vi "加标回收参数设置.vi"() -> ()   [LabVIEW 2016, in "质控单元V1.lvlib"]
panel:
  in  "显示详细日志":bool
  in  "布尔":bool
  in  "Tab Control 2":enum32{"氨氮", "总磷", "总氮", "高锰酸盐指数", "化学需氧量"}(tab)
  in  "启用":bool
  out "氨氮加标回收率":sgl caption="加标回收率" format="%#.2f"
  out "氨氮加标体积":sgl caption="加标体积" format="%#.4f"
  in  "氨氮母液浓度":sgl caption="母液浓度"
  in  "氨氮定容体积":sgl caption="定容体积"
  out "氨氮加标后水样浓度":sgl caption="加标后水样浓度" format="%#.4f"
  out "氨氮加标前水样浓度":sgl caption="加标前水样浓度" format="%#.4f"
  in  "氨氮量程":sgl caption="量程"
  in  "氨氮检出限":sgl caption="检出限"
  in  "启用 2":bool
  out "TP加标回收率":sgl caption="加标回收率" format="%#.2f"
  out "TP加标体积":sgl caption="加标体积" format="%#.4f"
  in  "TP母液浓度":sgl caption="母液浓度"
  in  "TP定容体积":sgl caption="定容体积"
  out "TP加标后水样浓度":sgl caption="加标后水样浓度" format="%#.4f"
  out "TP加标前水样浓度":sgl caption="加标前水样浓度" format="%#.4g"
  in  "TP量程":sgl caption="量程"
  in  "TP检出限":sgl caption="检出限"
  in  "启用 3":bool
  out "TN加标回收率":sgl caption="加标回收率" format="%#.2f"
  out "TN加标体积":sgl caption="加标体积" format="%#.4f"
  in  "TN母液浓度":sgl caption="母液浓度"
  in  "TN定容体积":sgl caption="定容体积"
  out "TN加标后水样浓度":sgl caption="加标后水样浓度" format="%#.4f"
  out "TN加标前水样浓度":sgl caption="加标前水样浓度" format="%#.4f"
  in  "TN量程":sgl caption="量程"
  in  "TN检出限":sgl caption="检出限"
  in  "启用 4":bool
  out "CODMn加标回收率":sgl caption="加标回收率" format="%#.2f"
  out "CODMn加标体积":sgl caption="加标体积" format="%#.4f"
  in  "CODMn母液浓度":sgl caption="母液浓度"
  in  "CODMn定容体积":sgl caption="定容体积"
  out "CODMn加标后水样浓度":sgl caption="加标后水样浓度" format="%#.4f"
  out "CODMn加标前水样浓度":sgl caption="加标前水样浓度" format="%#.4f"
  in  "CODMn量程":sgl caption="量程"
  in  "CODMn检出限":sgl caption="检出限"
  in  "启用 5":bool
  out "CODCr加标回收率":sgl caption="加标回收率" format="%#.2f"
  out "CODCr加标体积":sgl caption="加标体积" format="%#.4f"
  in  "CODCr母液浓度":sgl caption="母液浓度"
  in  "CODCr定容体积":sgl caption="定容体积"
  out "CODCr加标后水样浓度":sgl caption="加标后水样浓度" format="%#.4f"
  out "CODCr加标前水样浓度":sgl caption="加标前水样浓度" format="%#.4f"
  in  "CODCr量程":sgl caption="量程"
  in  "CODCr检出限":sgl caption="检出限"
  # "加标回收参数设置"
  # "加标回收参数"
  # "加标回收参数"
  # "加标回收参数"
  # "加标回收参数"
  # "加标回收参数"
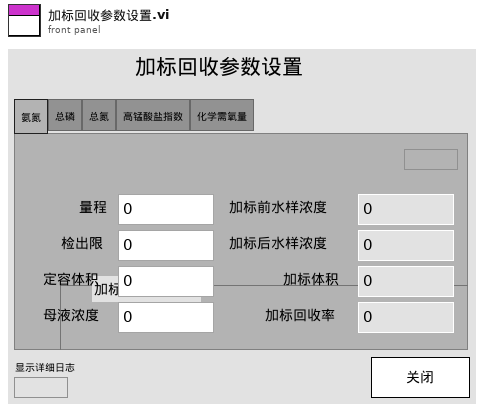
[diagram p1: front panel]
types:
  T1 = cluster{"量程":dbl, "检出限":dbl, "加标前水样浓度":dbl, "加标后水样浓度":dbl, "加标水杯定容体积":dbl, "加标母液浓度":dbl, "加标体积":dbl, "加标回收率":dbl}
  T2 = cluster{"氨氮":bool, "总磷":bool, "总氮":bool, "CODMn":bool, "CODCr":bool, "氨氮总磷":bool, "总磷总氮":bool}
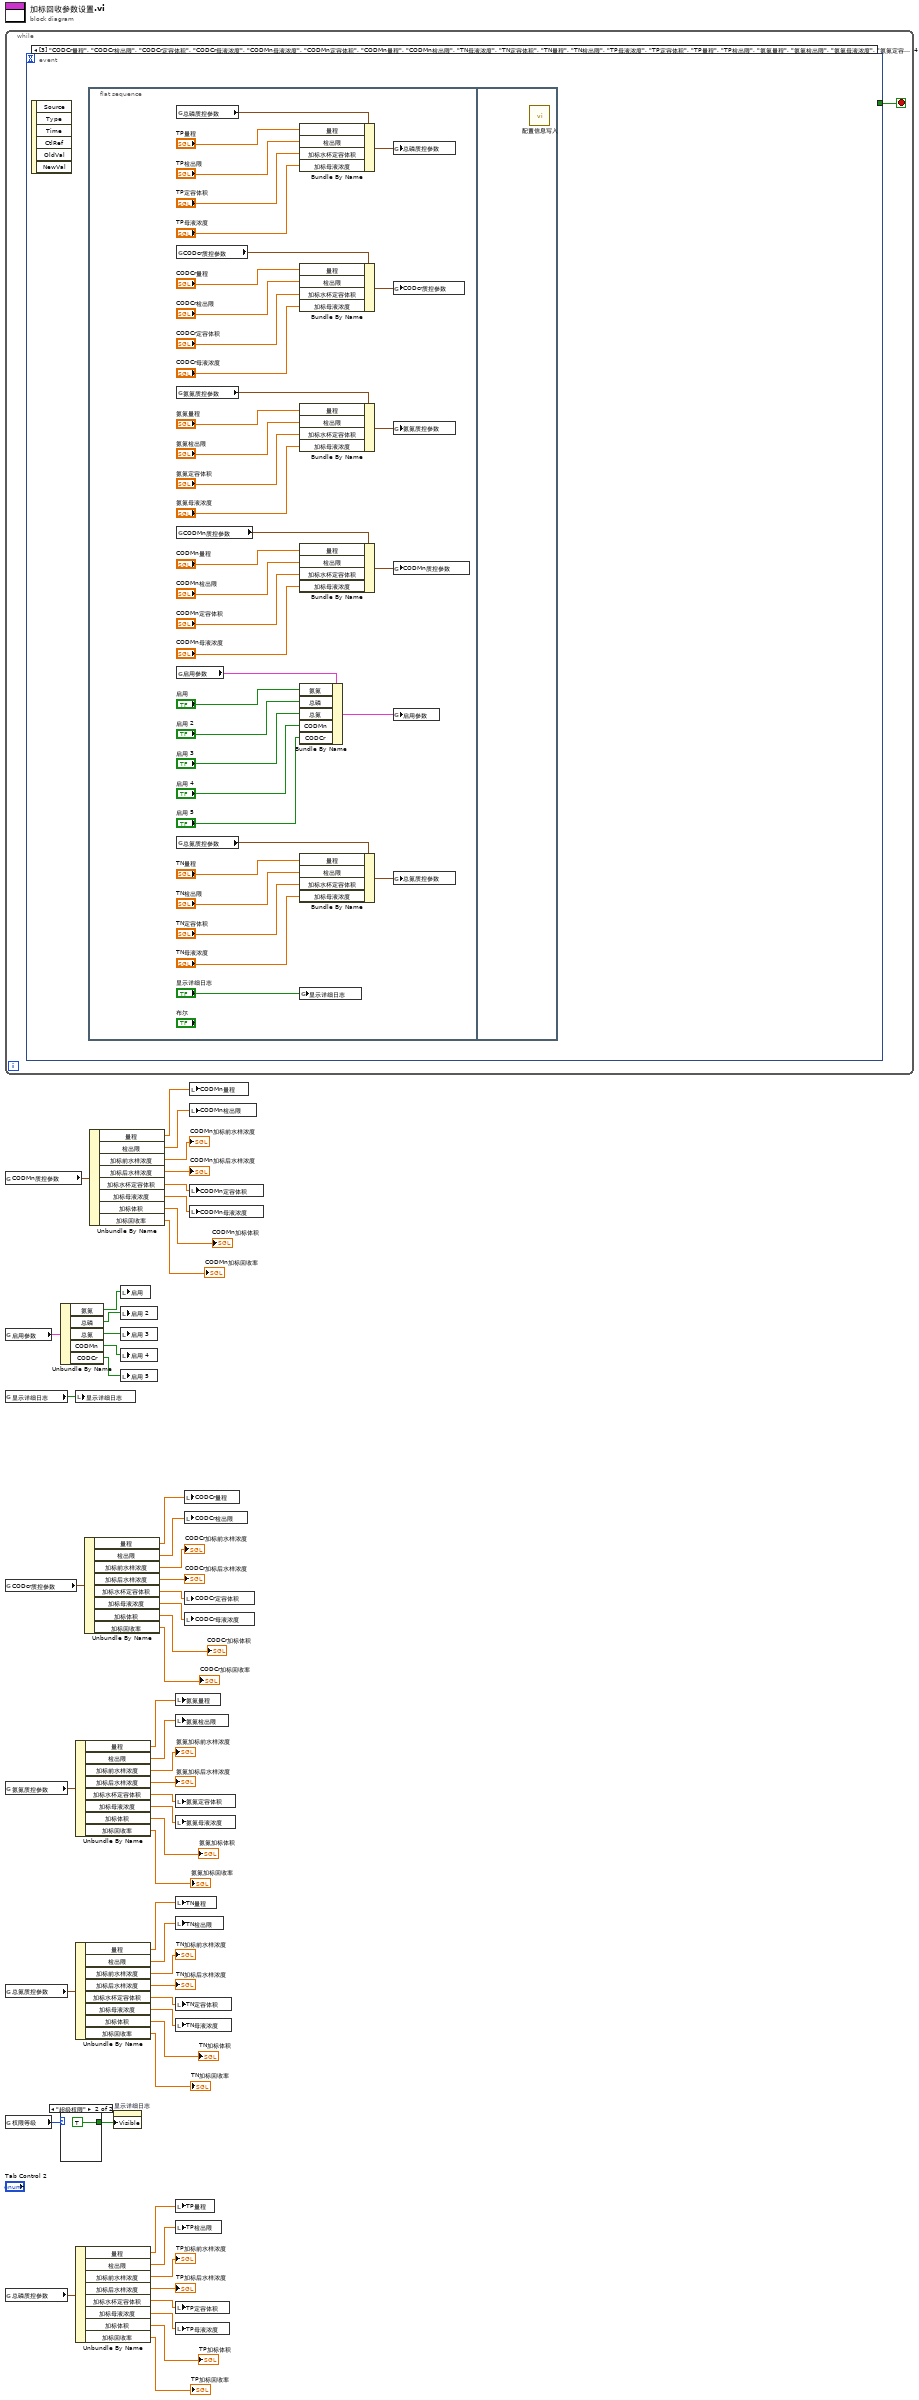
[diagram p0: block diagram]
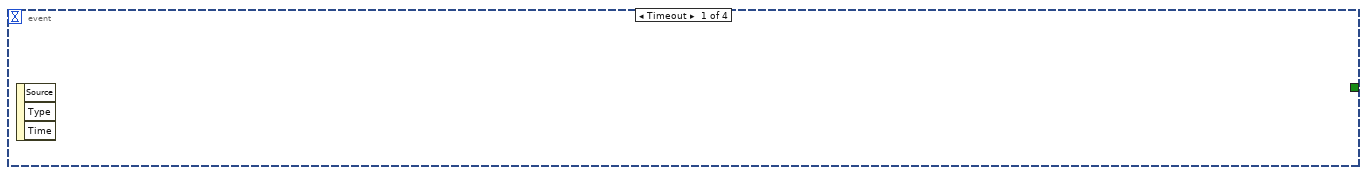
[diagram p3: hidden frame]
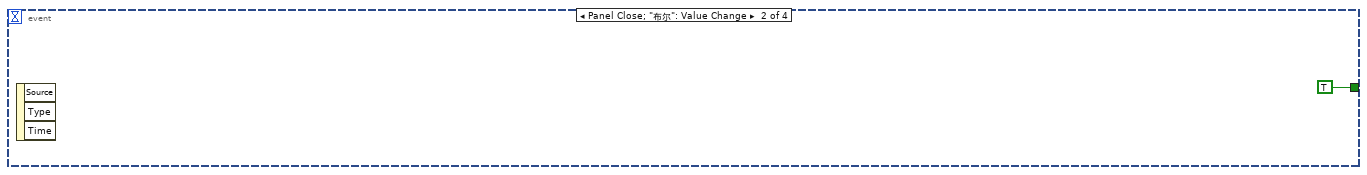
[diagram p4: hidden frame]
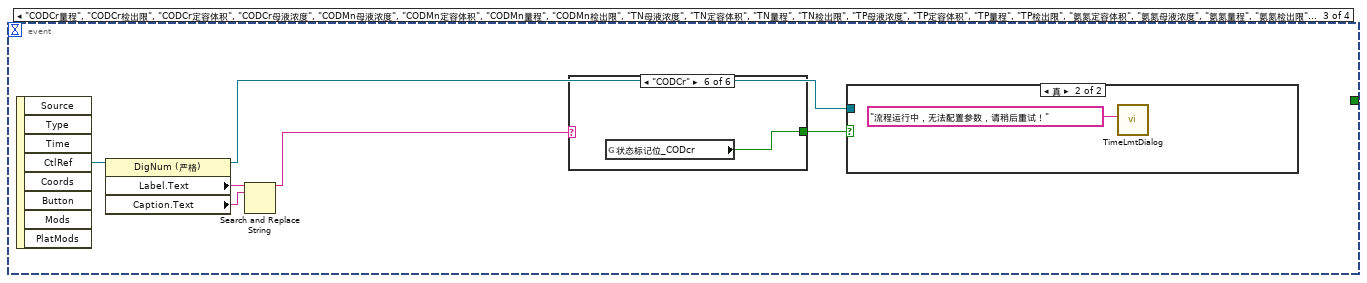
[diagram p5: hidden frame]
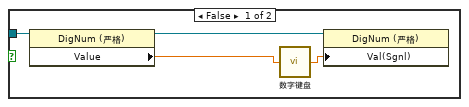
[diagram p6: hidden frame]
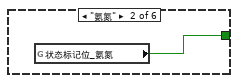
[diagram p8: hidden frame]
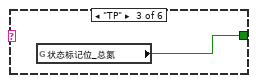
[diagram p9: hidden frame]
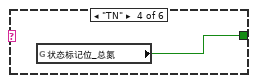
[diagram p10: hidden frame]
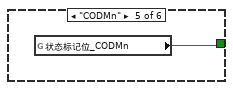
[diagram p11: hidden frame]
diagram:
  n1 = while {
    stop <- w55 stop-if-true
    n2 = event shown="[3] \"CODCr量程\", \"CODCr检出限\", \"CODCr定容体积\", \"CODCr母液浓度\", \"CODMn母液浓度\", \"CODMn定容体积\", \"CODMn量程\", \"CODMn检出限\", \"TN母液浓度\", \"TN定容体积\", \"TN量程\", \"TN检出限\", \"TP母液浓度\", \"TP定容体积\", \"TP量程\", \"TP检出限\", \"氨氮量程\", \"氨氮检出限\", \"氨氮母液浓度\", \"氨氮定容体积\", \"启用\", \"启用 2\", \"启用 3\", \"启用 4\", \"启用 5\", \"显示详细日志\": 值改变" {
      selector: _ -> [_ _ _ _]
      dyn-events: _ -> [_ _ _ _]
      timeout: _ -> [_ _ _ _]
      tunnel: [_ TRUE _ _] -> w55
      event Timeout {
        n3 = event-data() -> ()  [unwired: 1 in, 3 out]
      }
      event Panel Close; "布尔": Value Change {
        n4 = event-data() -> ()  [unwired: 1 in, 3 out]
      }
      event "CODCr量程", "CODCr检出限", "CODCr定容体积", "CODCr母液浓度", "CODMn母液浓度", "CODMn定容体积", "CODMn量程", "CODMn检出限", "TN母液浓度", "TN定容体积", "TN量程", "TN检出限", "TP母液浓度", "TP定容体积", "TP量程", "TP检出限", "氨氮定容体积", "氨氮母液浓度", "氨氮量程", "氨氮检出限": Mouse Down {
        n5 = event-data() -> ("CtlRef"=w62:refnum<vi>)  [unwired: 1 in, 7 out]
        n6 = property class="DigNum (严格)"(reference=w62) -> (reference out=w61:refnum<vi>, "Label.Text"=w60:string, "Caption.Text"=w59:string)  [unwired: 1 in, 1 out]
        n7 = Search and Replace String(input string=w60, search string=w59) -> (result string=w58:string)  [unwired: 6 in, 3 out]
        n8 = case shown="\"CODCr\"" w58 {
          tunnel: [_ w68 w69 w70 w71 w72] -> w57
          frame Default {
          }
          frame "氨氮" {
            n9 = global read "ZK非断电保存全局变量.vi" "状态标记位_氨氮"() -> (w68:bool)
          }
          frame "TP" {
            n10 = global read "ZK非断电保存全局变量.vi" "状态标记位_总氮"() -> (w69:bool)
          }
          frame "TN" {
            n11 = global read "ZK非断电保存全局变量.vi" "状态标记位_总氮"() -> (w70:bool)
          }
          frame "CODMn" {
            n12 = global read "ZK非断电保存全局变量.vi" "状态标记位_CODMn"() -> (w71:bool)
          }
          frame "CODCr" {
            n13 = global read "ZK非断电保存全局变量.vi" "状态标记位_CODcr"() -> (w72:bool)
          }
        }
        n14 = case shown="真" w57 {
          tunnel: w61 -> [w63 _]
          frame False {
            n15 = property class="DigNum (严格)"(reference=w63) -> (reference out=w65:refnum<vi>, "Value"=w66:sgl)  [unwired: 1 in, 1 out]
            n16 = call "数字键盘.vi"("OldNumber"=w66) -> ("NewNumber"=w64:sgl)
            n17 = property class="DigNum (严格)"(reference=w65, "Val(Sgnl)"=w64) -> ()  [unwired: 1 in, 2 out]
          }
          frame True {
            n18 = call "TimeLmtDialog.vi"("Infoin"="流程运行中，无法配置参数，请稍后重试！") -> ()  [unwired: 11 in]
          }
        }
      }
      event "CODCr量程", "CODCr检出限", "CODCr定容体积", "CODCr母液浓度", "CODMn母液浓度", "CODMn定容体积", "CODMn量程", "CODMn检出限", "TN母液浓度", "TN定容体积", "TN量程", "TN检出限", "TP母液浓度", "TP定容体积", "TP量程", "TP检出限", "氨氮量程", "氨氮检出限", "氨氮母液浓度", "氨氮定容体积", "启用", "启用 2", "启用 3", "启用 4", "启用 5", "显示详细日志": Value Change {
        n19 = event-data() -> ()  [unwired: 1 in, 6 out]
        n20 = flat-sequence {
          frame #0 {
            n21 = global read "ZK断电保存全局变量.vi" "总磷质控参数"() -> (w86:T1)
            n22 = global read "ZK断电保存全局变量.vi" "CODcr质控参数"() -> (w103:T1)
            n23 = global read "ZK断电保存全局变量.vi" "氨氮质控参数"() -> (w98:T1)
            n24 = global read "ZK断电保存全局变量.vi" "CODMn质控参数"() -> (w110:T1)
            n25 = global read "ZK断电保存全局变量.vi" "启用参数"() -> (w80:T2)
            n26 = global read "ZK断电保存全局变量.vi" "总氮质控参数"() -> (w91:T1)
            n27 = Bundle By Name(cluster=w86, "量程"="TP量程", "检出限"="TP检出限", "加标水杯定容体积"="TP定容体积", "加标母液浓度"="TP母液浓度") -> (w85:T1)
            n28 = Bundle By Name(cluster=w103, "量程"="CODCr量程", "检出限"="CODCr检出限", "加标水杯定容体积"="CODCr定容体积", "加标母液浓度"="CODCr母液浓度") -> (w104:T1)
            n29 = Bundle By Name(cluster=w98, "量程"="氨氮量程", "检出限"="氨氮检出限", "加标水杯定容体积"="氨氮定容体积", "加标母液浓度"="氨氮母液浓度") -> (w97:T1)
            n30 = Bundle By Name(cluster=w110, "量程"="CODMn量程", "检出限"="CODMn检出限", "加标水杯定容体积"="CODMn定容体积", "加标母液浓度"="CODMn母液浓度") -> (w109:T1)
            n31 = Bundle By Name(cluster=w80, "氨氮"="启用", "总磷"="启用 2", "总氮"="启用 3", "CODMn"="启用 4", "CODCr"="启用 5") -> (w79:T2)
            n32 = Bundle By Name(cluster=w91, "量程"="TN量程", "检出限"="TN检出限", "加标水杯定容体积"="TN定容体积", "加标母液浓度"="TN母液浓度") -> (w92:T1)
            n33 = global write "ZK断电保存全局变量.vi" "显示详细日志"("显示详细日志") -> ()
            n34 = global write "ZK断电保存全局变量.vi" "总磷质控参数"(w85) -> ()
            n35 = global write "ZK断电保存全局变量.vi" "CODcr质控参数"(w104) -> ()
            n36 = global write "ZK断电保存全局变量.vi" "氨氮质控参数"(w97) -> ()
            n37 = global write "ZK断电保存全局变量.vi" "CODMn质控参数"(w109) -> ()
            n38 = global write "ZK断电保存全局变量.vi" "启用参数"(w79) -> ()
            n39 = global write "ZK断电保存全局变量.vi" "总氮质控参数"(w92) -> ()
          }
          frame #1 {
            n40 = call "配置信息写入.vi"() -> ()  [unwired: 11 in, 1 out]
          }
        }
      }
    }
  }
  n41 = global read "ZK断电保存全局变量.vi" "CODMn质控参数"() -> (w54:T1)
  n42 = global read "ZK断电保存全局变量.vi" "启用参数"() -> (w9:T2)
  n43 = global read "ZK断电保存全局变量.vi" "显示详细日志"() -> (w3:bool)
  n44 = global read "ZK断电保存全局变量.vi" "CODcr质控参数"() -> (w45:T1)
  n45 = global read "ZK断电保存全局变量.vi" "氨氮质控参数"() -> (w36:T1)
  n46 = global read "ZK断电保存全局变量.vi" "总氮质控参数"() -> (w27:T1)
  n47 = global read "ZK非断电保存全局变量.vi" "权限等级"() -> (w2:enum16{"一级权限", "二级权限", "三级权限", "超级权限"})
  n48 = global read "ZK断电保存全局变量.vi" "总磷质控参数"() -> (w25:T1)
  n49 = Unbundle By Name(w9) -> ("氨氮"=w8:bool, "总磷"=w7:bool, "总氮"=w6:bool, "CODMn"=w5:bool, "CODCr"=w4:bool)
  n50 = case shown="\"超级权限\"" w2 {
    tunnel: [_ TRUE] -> w1
    frame "一级权限", Default {
    }
    frame "超级权限" {
    }
  }
  n51 = local write "显示详细日志"(w3) -> ()
  n52 = Unbundle By Name(w36) -> ("量程"=w31:dbl, "检出限"=w30:dbl, "加标前水样浓度"=→"氨氮加标前水样浓度":dbl, "加标后水样浓度"=→"氨氮加标后水样浓度":dbl, "加标水杯定容体积"=w29:dbl, "加标母液浓度"=w28:dbl, "加标体积"=→"氨氮加标体积":dbl, "加标回收率"=→"氨氮加标回收率":dbl)
  n53 = Unbundle By Name(w27) -> ("量程"=w13:dbl, "检出限"=w12:dbl, "加标前水样浓度"=→"TN加标前水样浓度":dbl, "加标后水样浓度"=→"TN加标后水样浓度":dbl, "加标水杯定容体积"=w11:dbl, "加标母液浓度"=w10:dbl, "加标体积"=→"TN加标体积":dbl, "加标回收率"=→"TN加标回收率":dbl)
  n54 = Unbundle By Name(w25) -> ("量程"=w17:dbl, "检出限"=w16:dbl, "加标前水样浓度"=→"TP加标前水样浓度":dbl, "加标后水样浓度"=→"TP加标后水样浓度":dbl, "加标水杯定容体积"=w15:dbl, "加标母液浓度"=w14:dbl, "加标体积"=→"TP加标体积":dbl, "加标回收率"=→"TP加标回收率":dbl)
  n55 = Unbundle By Name(w45) -> ("量程"=w40:dbl, "检出限"=w39:dbl, "加标前水样浓度"=→"CODCr加标前水样浓度":dbl, "加标后水样浓度"=→"CODCr加标后水样浓度":dbl, "加标水杯定容体积"=w38:dbl, "加标母液浓度"=w37:dbl, "加标体积"=→"CODCr加标体积":dbl, "加标回收率"=→"CODCr加标回收率":dbl)
  n56 = Unbundle By Name(w54) -> ("量程"=w49:dbl, "检出限"=w48:dbl, "加标前水样浓度"=→"CODMn加标前水样浓度":dbl, "加标后水样浓度"=→"CODMn加标后水样浓度":dbl, "加标水杯定容体积"=w47:dbl, "加标母液浓度"=w46:dbl, "加标体积"=→"CODMn加标体积":dbl, "加标回收率"=→"CODMn加标回收率":dbl)
  n57 = property on="显示详细日志" class="Bool (严格)"("Visible"=w1) -> ()  [unwired: 2 in, 2 out]
  n58 = local write "启用"(w8) -> ()
  n59 = local write "启用 2"(w7) -> ()
  n60 = local write "启用 3"(w6) -> ()
  n61 = local write "启用 4"(w5) -> ()
  n62 = local write "启用 5"(w4) -> ()
  n63 = local write "氨氮量程"(w31) -> ()
  n64 = local write "氨氮检出限"(w30) -> ()
  n65 = local write "氨氮定容体积"(w29) -> ()
  n66 = local write "氨氮母液浓度"(w28) -> ()
  n67 = local write "TN量程"(w13) -> ()
  n68 = local write "TN检出限"(w12) -> ()
  n69 = local write "TN定容体积"(w11) -> ()
  n70 = local write "TN母液浓度"(w10) -> ()
  n71 = local write "TP量程"(w17) -> ()
  n72 = local write "TP检出限"(w16) -> ()
  n73 = local write "TP定容体积"(w15) -> ()
  n74 = local write "TP母液浓度"(w14) -> ()
  n75 = local write "CODCr量程"(w40) -> ()
  n76 = local write "CODCr检出限"(w39) -> ()
  n77 = local write "CODCr定容体积"(w38) -> ()
  n78 = local write "CODCr母液浓度"(w37) -> ()
  n79 = local write "CODMn量程"(w49) -> ()
  n80 = local write "CODMn检出限"(w48) -> ()
  n81 = local write "CODMn定容体积"(w47) -> ()
  n82 = local write "CODMn母液浓度"(w46) -> ()
